vi "DAQmx Create Channel (CI-Pulse Width).vi"(0 "task in":refnum<k21>, 1 "maximum value":dbl=0.1 format="%.6f", 2 "minimum value":dbl=1e-06 format="%.6f", 5 "counter":tag, 7 "name to assign":string, 9 "units":i32(ring)=10364 items=["Seconds"=10364, "Ticks"=10304, "From Custom Scale"=10065], 11 "error in":errorcluster, 12 "custom scale name":tag, 13 "starting edge":i32(ring)=10280 items=["Rising"=10280, "Falling"=10171]) -> (4 "task out":refnum<k21>, 15 "error out":errorcluster)   [LabVIEW 2013]
doc: "Creates a channel to measure the width of a digital pulse. <B>starting edge</B> determines whether to measure a high pulse or low pulse. With the exception of devices that support multi-counter tasks, you can create only one counter input channel at a time with this VI because a task can contain only one counter input channel. To read from multiple counters simultaneously, use a separate task for each counter. Connect the input signal to the default input terminal of the counter unless you select a different input terminal."
uses:
  <resource>/objmgr/daqmx.rc
panel:
  # "input limits"
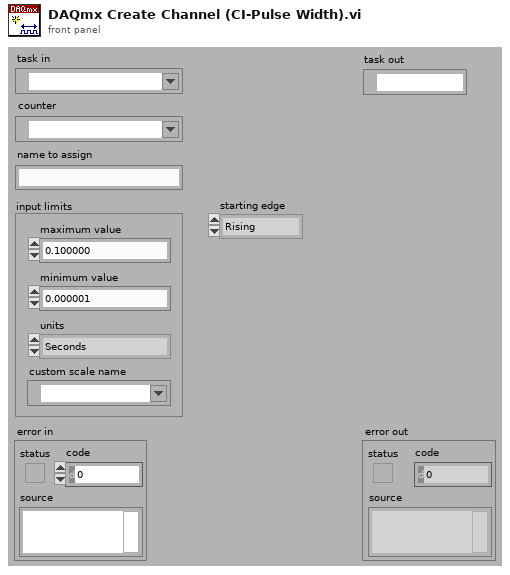
[diagram p1: front panel]
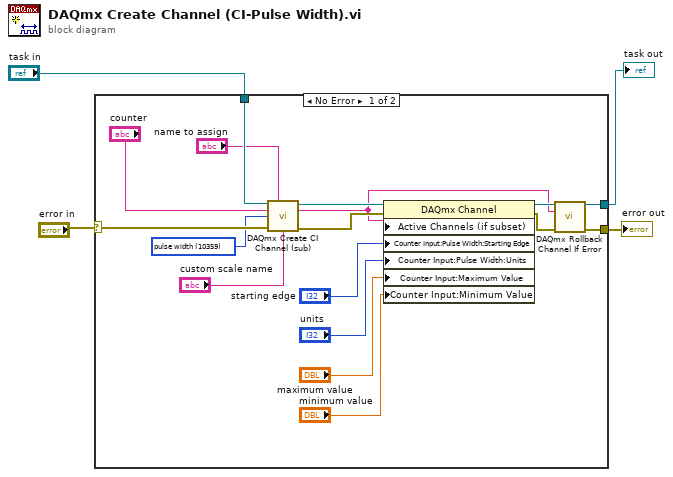
[diagram p0: block diagram]
diagram:
  n1 = case shown="No Error" "error in" {
    selector: "error in" -> [w19 w22]
    tunnel: "task in" -> [w21 w23]
    tunnel: [w8 w23] -> w2
    tunnel: [w7 w22] -> w1
    frame No Error {
      w12 = 10359 items=["count events"=10125, "frequency"=10179, "period"=10256, "pulse width"=10359, "semi period"=10289] ("measurement type")
      n2 = call "DAQmx Create CI Channel (sub).vi"("task in"=w21, "virtual channel name"="name to assign", "physical channel name"="counter", "measurement type"=w12, "error in"=w19, "custom scale"="custom scale name") -> ("task out"=w10:refnum<k21>, "channel names"=w5:string, "error out"=w18:errorcluster)  [unwired: 7 out]
      n3 = property class="DAQmx Channel"(reference=w10, error in=w18, "Active Channels (if subset)"=w5, "Counter Input:Pulse Width:Starting Edge"="starting edge", "Counter Input:Pulse Width:Units"="units", "Counter Input:Maximum Value"="maximum value", "Counter Input:Minimum Value"="minimum value") -> (reference out=w9:refnum<k21>, error out=w6:errorcluster)
      n4 = call "DAQmx Rollback Channel If Error.vi"("task in"=w9, "channel names"=w5, "error in"=w6) -> ("task out"=w8:refnum<k21>, "error out"=w7:errorcluster)  [unwired: 11 out]
    }
    frame Error {
    }
  }
  "error out" <- w1
  "task out" <- w2
